vi "DisconnectR.vi"(0 "RBD9103":T1, 5 "error in":errorcluster) -> (19 "error out":errorcluster)   [LabVIEW 2018]
uses:
  RBD9103.ctl
  GenericDataEvent/GenericEvent.ctl
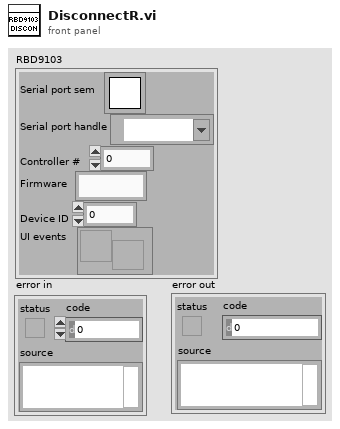
[diagram p1: front panel]
types:
  T1 = typedef "RBD9103.ctl" = cluster{"Serial port sem":T2, "Serial port handle":refnum<visa-resource-name>, "Controller #":u8, "Firmware":string, "Device ID":i32, "UI events":T3}
  T2 = typedef "Semaphore RefNum" = refnum<k1>
  T3 = typedef "GenericEvent.ctl" = refnum<user-event>
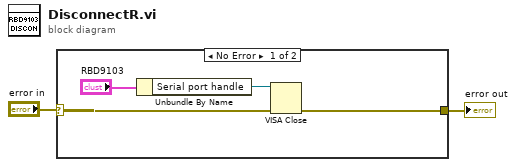
[diagram p0: block diagram]
diagram:
  n1 = case shown="No Error" "error in" {
    selector: "error in" -> [w5 w7]
    tunnel: [w3 w7] -> w1
    frame No Error {
      n2 = Unbundle By Name("RBD9103") -> ("Serial port handle"=w6:refnum<visa-resource-name>)
      n3 = VISA Close(VISA resource name=w6, error in (no error)=w5) -> (error out=w3:errorcluster)
    }
    frame Error {
    }
  }
  "error out" <- w1
